vi "DamnYankeeHindbrainSense.vi"(9 "Notifier References":T5, 10 "Data Queue clusters":T4, 11 "IO Cluster":T1) -> (0 "error out":errorcluster)   [LabVIEW 2013]
doc: "This VI grabs sensor data from the MyRIO I/O ports and packages it into queues. These queues go directly to HB Sense, which filters the data and writes it to notifiers.\n\nIF ONE SENSOR TAKES MUCH LONGER THAN OTHER SENSORS IT SHOULD BE SPLIT OUT INTO A SEPARATE WHILE LOOP. We don't know about speeds yet.\n\nEric Schneider, April 2014"
uses:
  Data/TypeDefs/Notifiers.ctl
  Data/TypeDefs/UTM Location.ctl
  Data/TypeDefs/Sail Set Suggestions.ctl
  Data/TypeDefs/Rudder Set Suggestions.ctl
  Data/TypeDefs/OverrideInformation.ctl
  Data/TypeDefs/OverrideMode.ctl
  Data/TypeDefs/MotorSetup.ctl
  Data/TypeDefs/DynamixelSetupInfo.ctl
  Data/TypeDefs/AirmarStatus.ctl
  Data/TypeDefs/HardwareOnline.ctl
  Data/TypeDefs/DynamixelCycleTracker.ctl
  Data/TypeDefs/RC Input Values.ctl
  Classes/Waypoint/Waypoint.lvclass
  Data/TypeDefs/GPS-Compass Queue Cluster.ctl
  Data/TypeDefs/WindData Queue Cluster.ctl
  Data/TypeDefs/DamnYankeeIOPorts.ctl
panel:
  out "Measured wind angle":dbl
  # "Debugging information"
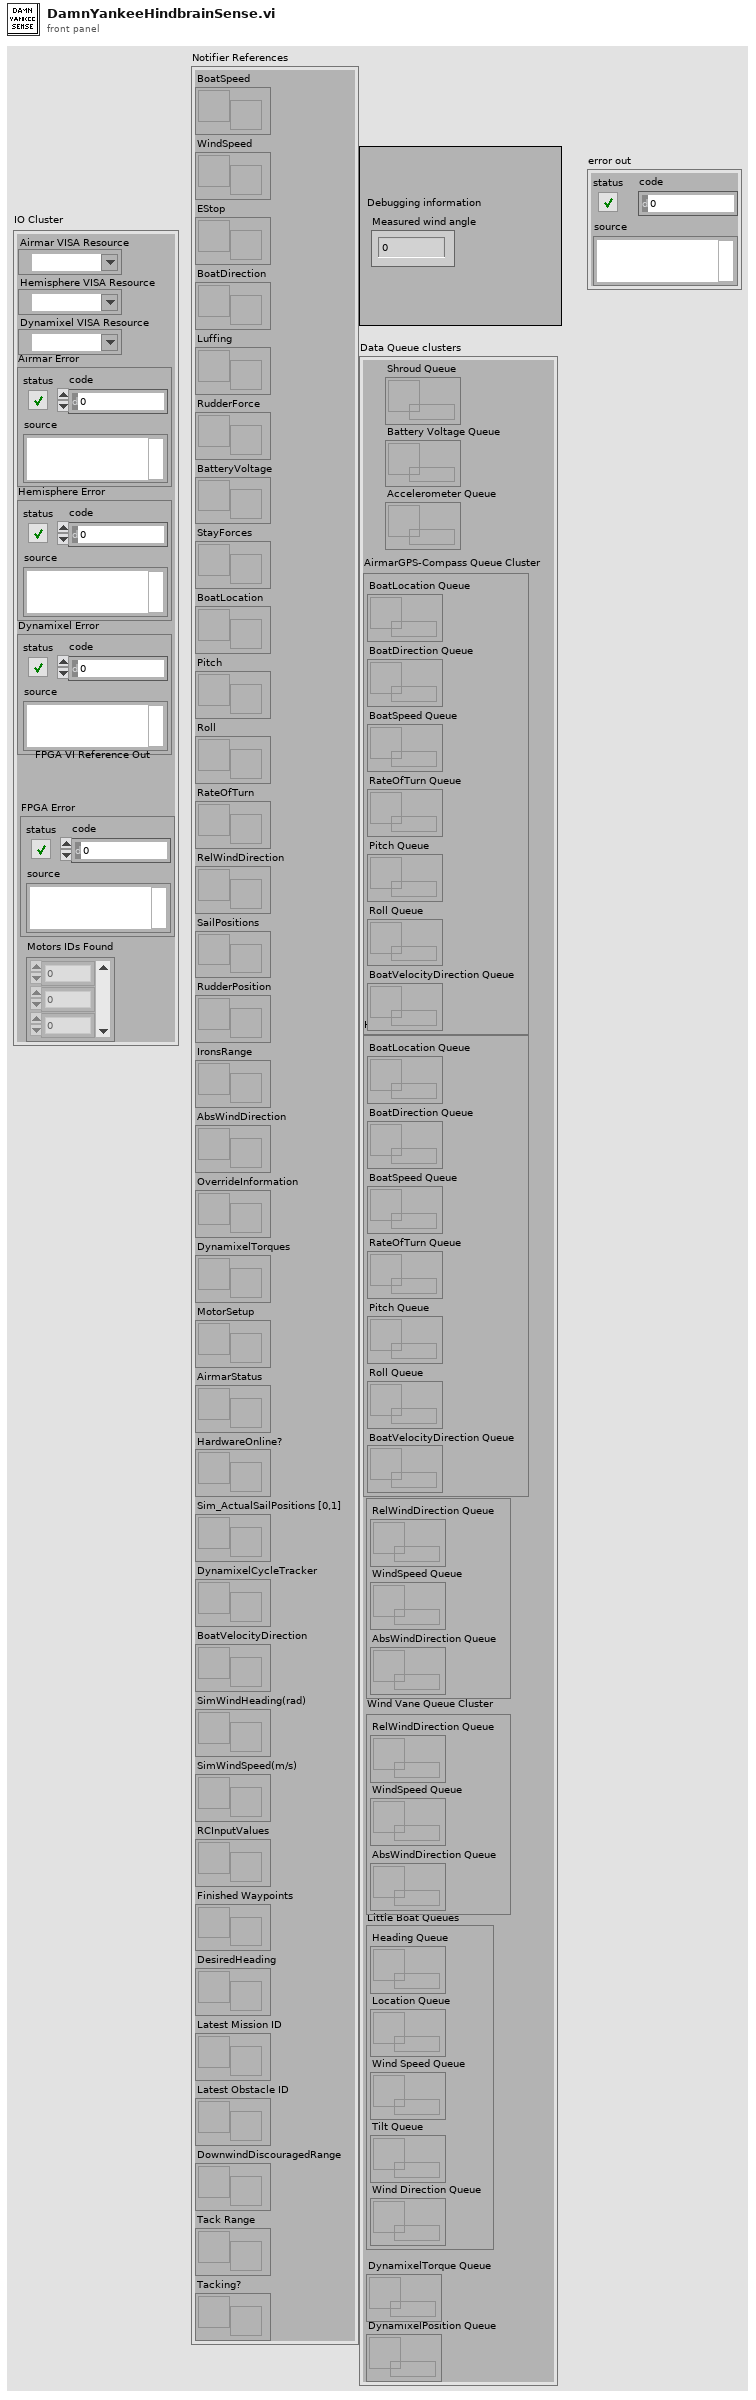
[diagram p1: front panel]
types:
  T1 = typedef "DamnYankeeIOPorts.ctl" = cluster{"Airmar VISA Resource":refnum<visa-resource-name>, "Hemisphere VISA Resource":refnum<visa-resource-name>, "Dynamixel VISA Resource":refnum<visa-resource-name>, "Airmar Error":errorcluster, "Hemisphere Error":errorcluster, "Dynamixel Error":errorcluster, "FPGA Error":errorcluster, "FPGA VI Reference Out":refnum<k20>, "Motors IDs Found":u8[]}
  T2 = typedef "GPS-Compass Queue Cluster.ctl" = cluster{"BoatLocation Queue":refnum<queue>, "BoatDirection Queue":refnum<queue>, "BoatSpeed Queue":refnum<queue>, "RateOfTurn Queue":refnum<queue>, "Pitch Queue":refnum<queue>, "Roll Queue":refnum<queue>, "BoatVelocityDirection Queue ":refnum<queue>}
  T3 = typedef "WindData Queue Cluster.ctl" = cluster{"RelWindDirection Queue":refnum<queue>, "WindSpeed Queue":refnum<queue>, "AbsWindDirection Queue":refnum<queue>}
  T4 = cluster{"Shroud Queue":refnum<queue>, "Battery Voltage Queue":refnum<queue>, "Accelerometer Queue":refnum<queue>, "AirmarGPS-Compass Queue Cluster":T2, "Hemisphere Queue Cluster":T2, "Airmar Wind Queue Cluster":T3, "Wind Vane Queue Cluster":T3, "Little Boat Queues":cluster{"Heading Queue":refnum<queue>, "Location Queue":refnum<queue>, "Wind Speed Queue":refnum<queue>, "Tilt Queue":refnum<queue>, "Wind Direction Queue":refnum<queue>}, "DynamixelTorque Queue":refnum<queue>, "DynamixelPosition Queue":refnum<queue>}
  T5 = typedef "Notifiers.ctl" = cluster{"BoatSpeed":refnum<notifier>, "WindSpeed":refnum<notifier>, "EStop":refnum<notifier>, "BoatDirection":refnum<notifier>, "Luffing":refnum<notifier>, "RudderForce":refnum<notifier>, "BatteryVoltage":refnum<notifier>, "StayForces":refnum<notifier>, "BoatLocation":refnum<notifier>, "Pitch":refnum<notifier>, "Roll":refnum<notifier>, "RateOfTurn":refnum<notifier>, "RelWindDirection":refnum<notifier>, "SailPositions":refnum<notifier>, "RudderPosition":refnum<notifier>, "IronsRange":refnum<notifier>, "AbsWindDirection":refnum<notifier>, "OverrideInformation":refnum<notifier>, "DynamixelTorques":refnum<notifier>, "MotorSetup":refnum<notifier>, "AirmarStatus":refnum<notifier>, "HardwareOnline?":refnum<notifier>, "Sim_ActualSailPositions [0,1]":refnum<notifier>, "DynamixelCycleTracker":refnum<notifier>, "BoatVelocityDirection":refnum<notifier>, "SimWindHeading(rad)":refnum<notifier>, "SimWindSpeed(m/s)":refnum<notifier>, "RCInputValues":refnum<notifier>, "Finished Waypoints":refnum<notifier>, "DesiredHeading":refnum<notifier>, "Latest Mission ID":refnum<notifier>, "Latest Obstacle ID":refnum<notifier>, "DownwindDiscouragedRange":refnum<notifier>, "Tack Range":refnum<notifier>, "Tacking?":refnum<notifier>}
  T6 = typedef "HardwareOnline.ctl" = cluster{"AirmarOnline":bool, "WindvaneOnline":bool, "HemisphereOnline":bool, "StayForceOnline":bool, "BatteryVoltageOnline":bool, "AccelerometerOnline":bool, "MainDynamixel Online":bool, "JibDynamixel Online":bool, "RudderDynamixel Online":bool}
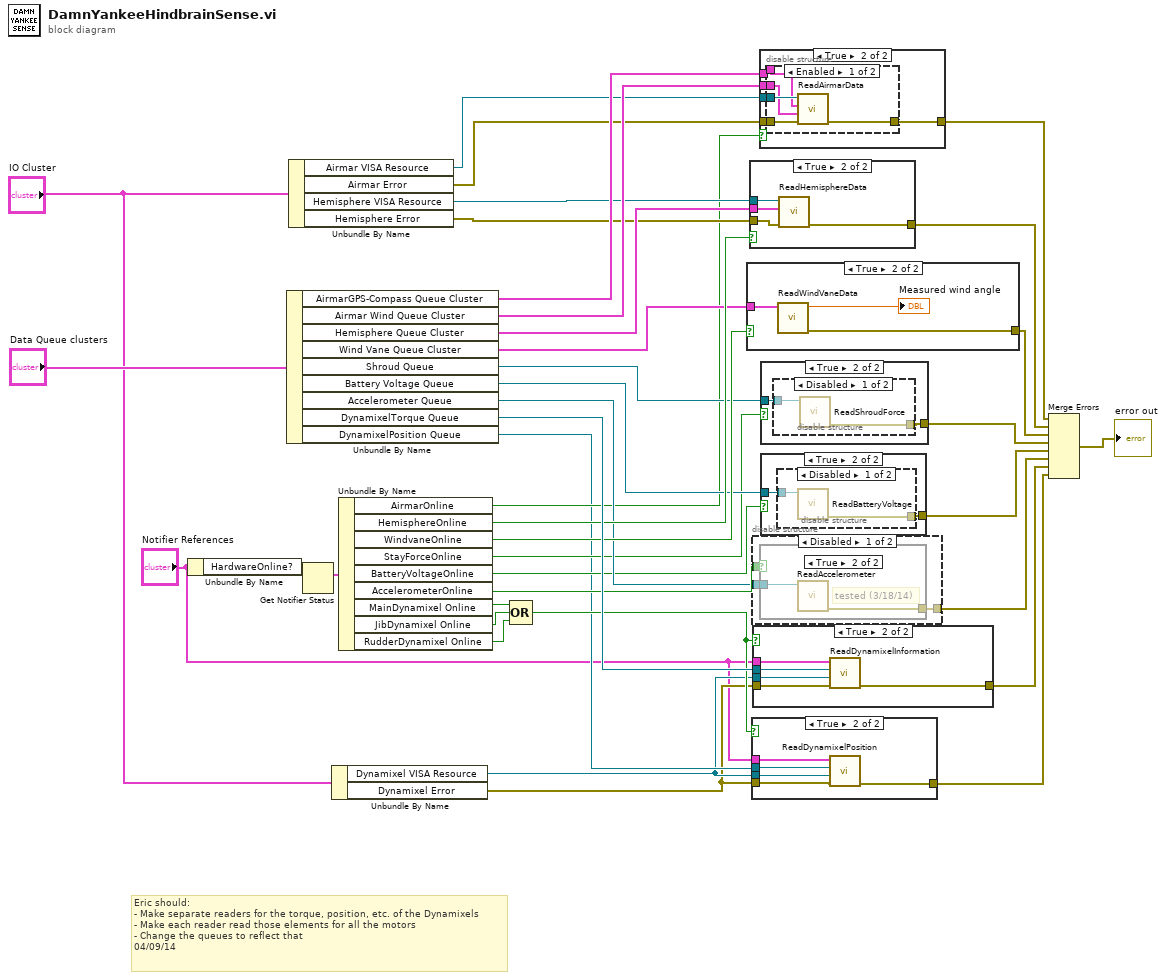
[diagram p0: block diagram]
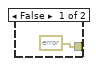
[diagram p2: hidden frame]
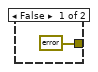
[diagram p6: hidden frame]
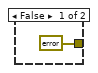
[diagram p8: hidden frame]
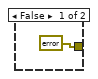
[diagram p10: hidden frame]
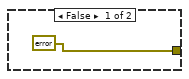
[diagram p11: hidden frame]
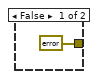
[diagram p12: hidden frame]
diagram:
  # "Eric should:\n- Make separate readers for the torque, position, etc. of the Dynamixels\n- Make each reader read those elements for all the motors\n- Change the queues to reflect that\n04/09/14"
  n1 = Unbundle By Name("Notifier References") -> ("HardwareOnline?"=w15:refnum<notifier>)
  n2 = Unbundle By Name("Data Queue clusters") -> ("AirmarGPS-Compass Queue Cluster"=w26:T2, "Airmar Wind Queue Cluster"=w27:T3, "Hemisphere Queue Cluster"=w28:T2, "Wind Vane Queue Cluster"=w29:T3, "Shroud Queue"=w22:refnum<queue>, "Battery Voltage Queue"=w24:refnum<queue>, "Accelerometer Queue"=w25:refnum<queue>, "DynamixelTorque Queue"=w39:refnum<queue>, "DynamixelPosition Queue"=w7:refnum<queue>)
  n3 = Unbundle By Name("IO Cluster") -> ("Airmar VISA Resource"=w17:refnum<visa-resource-name>, "Airmar Error"=w18:errorcluster, "Hemisphere VISA Resource"=w19:refnum<visa-resource-name>, "Hemisphere Error"=w20:errorcluster)
  n4 = Get Notifier Status(notifier=w15) -> (current notification=w14:T6)  [unwired: 1 in, 4 out]
  n5 = Unbundle By Name("IO Cluster") -> ("Dynamixel VISA Resource"=w6:refnum<visa-resource-name>, "Dynamixel Error"=w5:errorcluster)
  n6 = Unbundle By Name(w14) -> ("AirmarOnline"=w16:bool, "HemisphereOnline"=w31:bool, "WindvaneOnline"=w30:bool, "StayForceOnline"=w21:bool, "BatteryVoltageOnline"=w23:bool, "AccelerometerOnline"=w32:bool, "MainDynamixel Online"=w12:bool, "JibDynamixel Online"=w11:bool, "RudderDynamixel Online"=w10:bool)
  n7 = Compound Arithmetic op=OR(w12, w11, w10) -> (w8:bool)
  n8 = case shown="True" w30 {
    tunnel: [errorcluster {"status"=FALSE, "code"=0, "source"=""} ("error out") w43] -> w36
    tunnel: w29 -> [_ w42]
    frame False {
    }
    frame True {
      n9 = call "ReadWindVaneData.vi"("Wind Vane Queue Cluster"=w42) -> ("error out"=w43:errorcluster, "Measured wind angle"=→"Measured wind angle":dbl)  [unwired: 8 in, 1 out]
    }
  }
  n10 = case shown="True" w31 {
    tunnel: [errorcluster {"status"=FALSE, "code"=0, "source"=""} ("Error out") w48] -> w37
    tunnel: w19 -> [_ w47]
    tunnel: w20 -> [_ w46]
    tunnel: w28 -> [_ w45]
    frame False {
    }
    frame True {
      n11 = call "ReadHemisphereData.vi"("Error in"=w46, "Hemisphere Queue Cluster"=w45, "VISA UART port"=w47) -> ("Error out"=w48:errorcluster)  [unwired: 6 in, 2 out]
    }
  }
  n12 = case shown="True" w8 {
    tunnel: w7 -> [_ w54]
    tunnel: w6 -> [_ w53]
    tunnel: w5 -> [w49 w52]
    tunnel: "Notifier References" -> [_ w51]
    tunnel: [w49 w50] -> w3
    frame False {
    }
    frame True {
      n13 = call "ReadDynamixelPosition.vi"("error in (no error)"=w52, "VISA resource name"=w53, "DynamixelPositions Queue"=w54, "Notifier References"=w51) -> ("error out"=w50:errorcluster)  [unwired: 6 in, 1 out]
    }
  }
  n14 = disable-structure shown="Disabled" {
    disable-tunnel: [w57 _] -> w33
    disable-tunnel: w32 -> [w56 _]
    disable-tunnel: w25 -> [w55 _]
    frame Disabled {
      n15 = case shown="True" w56 {
        tunnel: [errorcluster {"status"=FALSE, "code"=0, "source"=""} ("error out") w60] -> w57
        tunnel: w55 -> [_ w59]
        frame False {
        }
        frame True {
          # "tested (3/18/14)"
          n16 = call "ReadAccelerometer.vi"("Accelerometer Queue"=w59) -> ("error out"=w60:errorcluster)  [unwired: 10 in]
        }
      }
    }
    frame Enabled {
    }
  }
  n17 = case shown="True" w8 {
    tunnel: w6 -> [_ w64]
    tunnel: w39 -> [_ w65]
    tunnel: w5 -> [w61 w63]
    tunnel: "Notifier References" -> [_ w66]
    tunnel: [w61 w62] -> w2
    frame False {
    }
    frame True {
      n18 = call "ReadDynamixelInformation.vi"("error in (no error)"=w63, "VISA resource name"=w64, "DynamixelTorque Queue"=w65, "Notifier References"=w66) -> ("error out"=w62:errorcluster)  [unwired: 6 in, 1 out]
    }
  }
  n19 = case shown="True" w16 {
    tunnel: w17 -> [_ w72]
    tunnel: w26 -> [_ w69]
    tunnel: w18 -> [_ w71]
    tunnel: [errorcluster {"status"=FALSE, "code"=0, "source"=""} ("Error out") w70] -> w38
    tunnel: w27 -> [_ w68]
    frame False {
    }
    frame True {
      n20 = disable-structure shown="Enabled" {
        disable-tunnel: w72 -> [w77 _]
        disable-tunnel: w71 -> [w76 _]
        disable-tunnel: [w75 _] -> w70
        disable-tunnel: w69 -> [w74 _]
        disable-tunnel: w68 -> [w73 _]
        frame Enabled {
          n21 = call "ReadAirmarData.vi"("Error in"=w76, "Airmar Wind Queue Cluster"=w73, "AirmarGPS-Compass Queue Cluster"=w74, "VISA UART port"=w77) -> ("Error out"=w75:errorcluster)  [unwired: 6 in, 1 out]
        }
        frame Disabled {
        }
      }
    }
  }
  n22 = case shown="True" w21 {
    tunnel: w22 -> [_ w80]
    tunnel: [errorcluster {"status"=FALSE, "code"=0, "source"=""} ("error out") w79] -> w35
    frame False {
    }
    frame True {
      n23 = disable-structure shown="Disabled" {
        disable-tunnel: w80 -> [w82 _]
        disable-tunnel: [w81 _] -> w79
        frame Disabled {
          n24 = call "ReadShroudForce.vi"("Queue in"=w82) -> ("error out"=w81:errorcluster)  [unwired: 9 in, 1 out]
        }
        frame Enabled {
        }
      }
    }
  }
  n25 = case shown="True" w23 {
    tunnel: w24 -> [_ w85]
    tunnel: [errorcluster {"status"=FALSE, "code"=0, "source"=""} ("error out") w84] -> w34
    frame False {
    }
    frame True {
      n26 = disable-structure shown="Disabled" {
        disable-tunnel: w85 -> [w87 _]
        disable-tunnel: [w86 _] -> w84
        frame Disabled {
          n27 = call "ReadBatteryVoltage.vi"("Queue in"=w87) -> ("error out"=w86:errorcluster)  [unwired: 9 in, 1 out]
        }
        frame Enabled {
        }
      }
    }
  }
  n28 = Merge Errors "Merge Errors"(w38, w37, w36, w35, w34, w33, w2, w3) -> (→"error out":errorcluster)
